vi "Binary_SpectroscopyFile-Close.vi"(8 "error in":errorcluster, 11 "File ref":refnum<file>) -> (0 "error out":errorcluster)   [LabVIEW 2017, in "Nanonis Prog Interface.lvlib"]
doc: "<b>Closes an open binary file.</b>\n\n- Nanonis Programming Interface-"
uses:
  Nanonis Prog Interface.lvlib
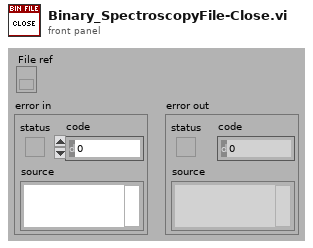
[diagram p1: front panel]
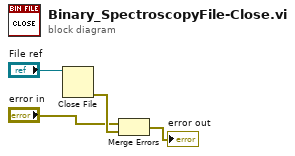
[diagram p0: block diagram]
diagram:
  n1 = Close File(refnum="File ref") -> (error out=w3:errorcluster)  [unwired: 1 in, 1 out]
  n2 = Merge Errors("error in", w3) -> (→"error out":errorcluster)
